vi "nanomsg_libpath.vi"() -> (0 "path":path)   [LabVIEW 2014, in "nanomsg.lvlib"]
doc: "Returns an absolute path to the LVZMQ shared library on the host system."
uses:
  nanomsg.lvlib
panel:
  # "NN"
  # "labview"
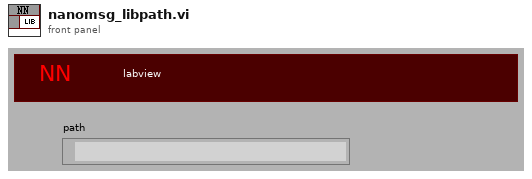
[diagram p1: front panel]
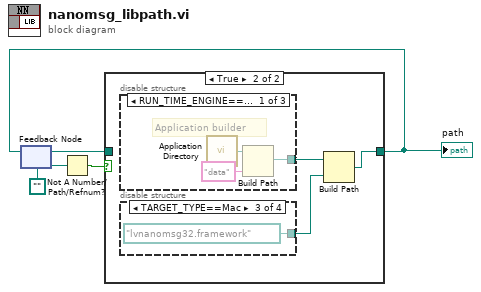
[diagram p0: block diagram]
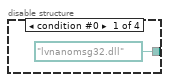
[diagram p3: hidden frame]
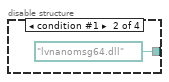
[diagram p4: hidden frame]
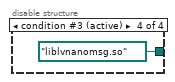
[diagram p5: hidden frame]
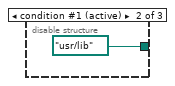
[diagram p6: hidden frame]
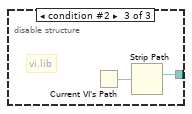
[diagram p7: hidden frame]
diagram:
  n1 = feedback #1(path "") -> (w2:path)
  n2 = Not A Number/Path/Refnum?(number/path/refnum=w2) -> (NaN/Path/Refnum?=w3:bool)
  n3 = case shown="True" w3 {
    tunnel: w2 -> [w5 _]
    tunnel: [w5 w6] -> w1
    frame False {
    }
    frame True {
      n4 = disable-structure shown="RUN_TIME_ENGINE==True" {
        disable-tunnel: [w15 path "/usr/lib" w18] -> w8
        frame condition #0 {
          # "Application builder"
          n5 = call <vilib>:"Application Directory.vi"() -> ("Application Directory"=w13:path)
          n6 = Build Path(base path=w13, name or relative path="data") -> (appended path=w15:path)
        }
        frame condition #1 (active) {
        }
        frame condition #2 {
          # "vi.lib"
          n7 = Current VI's Path() -> (path=w17:path)
          n8 = Strip Path(path=w17) -> (stripped path=w18:path)  [unwired: 1 out]
        }
      }
      n9 = disable-structure shown="TARGET_TYPE==Mac" {
        disable-tunnel: [path "lvnanomsg32.dll" ("appended path") path "lvnanomsg64.dll" ("appended path") path "lvnanomsg32.framework" ("appended path") path "liblvnanomsg.so" ("appended path")] -> w7
        frame condition #0 {
        }
        frame condition #1 {
        }
        frame condition #2 {
        }
        frame condition #3 (active) {
        }
      }
      n10 = Build Path(base path=w8, name or relative path=w7) -> (appended path=w6:path)
    }
  }
  "path" <- w1
  n11 = feedback-in #1(w1) -> ()
